vi "Cal Interpolation_3.vi"() -> ()   [LabVIEW 2018]
doc: "This example shows the operation of the 1D interpolation VI using three selectable test sets."
uses:
  <vilib>/Utility/file.llb/Read From Spreadsheet File (DBL).vi
  <vilib>/gmath/NI_Gmath.lvlib
panel:
  in  "file path (dialog if empty)":path=path "C:/IdtATE/Utilities/Calibration  Files/MIXER_TEST_032411_1939.csv"
  in  "y":dbl=201.0
  in  "all rows":dbl[][](array[numeric])=[[50000000.0, 100000000.0, 150000000.0, 200000000.0, 250000000.0, 300000000.0, 350000000.0, 400000000.0, 450000000.0, 500000000.0, 550000000.0, 600000000.0, 650000000.0, 700000000.0, 750000000.0, 800000000.0, 850000000.0, 900000000.0, 950000000.0, 1000000000.0, 1050000000.0, 1100000000.0, 1150000000.0, 1200000000.0, 1250000000.0, 1300000000.0, 1350000000.0, 1400000000.0, 1450000000.0, 1500000000.0, 1550000000.0, 1600000000.0, 1650000000.0, 1700000000.0, 1750000000.0, 1800000000.0, 1850000000.0, 1900000000.0, 1950000000.0, 2000000000.0, 2050000000.0, 2100000000.0, 2150000000.0, 2200000000.0, 2250000000.0, 2300000000.0, 2350000000.0, 2400000000.0, 2450000000.0, 2500000000.0, 2550000000.0, 2600000000.0, 2650000000.0, 2700000000.0, 2750000000.0, 2800000000.0, 2850000000.0, 2900000000.0, 2950000000.0, 3000000000.0], [-0.08, -0.16, -0.21, -0.23, -0.24, -0.28, -0.3, -0.34, -0.33, -0.31, -0.38, -0.37, -0.42, -0.39, -0.48, -0.41, -0.45, -0.41, -0.46, -0.48, -0.53, -0.57, -0.58, -0.65, -0.6, -0.71, -0.66, -0.77, -0.68, -0.78, -0.76, -0.88, -0.81, -0.83, -0.87, -0.83, -0.97, -0.81, -0.92, -0.79, -1.11, -0.76, -0.94, -0.98, -1.08, -0.9, -0.89, -1.14, -1.07, -1.25, -0.93, -1.25, -0.97, -1.38, -1.03, -1.17, -1.06, -1.21, -1.13, -0.98], [-6.65, -6.76, -6.93, -7.18, -7.18, -7.1, -7.38, -7.15, -7.28, -7.26, -7.24, -7.2, -7.36, -7.25, -7.49, -7.47, -7.53, -7.51, -7.88, -7.68, -7.97, -7.71, -7.89, -7.81, -7.91, -7.86, -7.94, -7.9, -7.97, -8.04, -8.08, -8.0, -8.12, -8.12, -8.29, -8.21, -8.41, -8.33, -8.43, -8.28, -8.91, -8.32, -8.78, -8.53, -8.99, -8.69, -8.98, -8.66, -9.24, -8.98, -8.95, -9.08, -9.02, -9.57, -9.73, -10.52, -10.26, -12.76, -13.4, -16.45], [-6.86, -6.86, -6.91, -7.31, -7.13, -7.12, -7.41, -7.13, -7.26, -7.16, -7.21, -7.16, -7.28, -7.19, -7.36, -7.35, -7.47, -7.41, -7.71, -7.57, -7.84, -7.64, -7.81, -7.77, -7.76, -7.89, -7.87, -7.94, -7.84, -8.05, -8.02, -8.06, -8.05, -8.14, -8.3, -8.19, -8.41, -8.36, -8.48, -8.27, -8.95, -8.31, -8.81, -8.49, -8.91, -8.64, -8.83, -8.49, -9.03, -8.8, -8.69, -8.97, -8.8, -9.38, -9.57, -10.78, -10.64, -12.82, -14.4, -17.28], [-0.19, -0.304, -0.304, -0.351, -0.339, -0.296, -0.371, -0.336, -0.432, -0.473, -0.503, -0.432, -0.446, -0.458, -0.627, -0.623, -0.587, -0.637, -0.778, -0.751, -0.707, -0.637, -0.654, -0.623, -0.707, -0.721, -0.778, -0.694, -0.707, -0.821, -0.991, -0.963, -0.778, -0.666, -0.749, -0.963, -1.093, -0.934, -0.877, -0.877, -1.05, -1.056, -0.892, -0.764, -0.877, -1.124, -1.272, -1.166, -1.05, -1.006, -1.008, -1.256, -1.345, -1.05, -1.008, -1.333, -1.516, -1.087, -1.124, -1.331]]
  in  "Freq Select":dbl=41000000.0
  out "Last Ofs Value":dbl=-0.07
  out "Next Ofs Value":dbl=-0.09
  out "Orig Ofs Data":dbl[](array[numeric])=[-0.07, -0.09, -0.13, -0.11, -0.14, -0.19, -0.14, -0.13, -0.21, -0.17, -0.19, -0.24, -0.26, -0.23, -0.25, -0.32, -0.32, -0.31, -0.3, -0.26, -0.27, -0.3, -0.28, -0.25, -0.34, -0.37, -0.34, -0.33, -0.35, -0.31, -0.36, -0.42, -0.36, -0.35, -0.42, -0.46, -0.39, -0.39, -0.39, -0.33, -0.35, -0.42, -0.39, -0.37, -0.39, -0.39, -0.36, -0.41, -0.46, -0.45, -0.48, -0.51, -0.54, -0.53, -0.52, -0.54, -0.53, -0.6, -0.6, -0.52, -0.59, -0.61, -0.57, -0.65, -0.67, -0.62, -0.61, -0.65, -0.68, -0.62, -0.67, -0.68, -0.66, -0.74, -0.78, -0.71, -0.69, -0.74, -0.77, -0.75, -0.8, -0.76, -0.73, -0.82, -0.84, -0.79, -0.74, -0.75, -0.75, -0.8, -0.9, -0.87, -0.74, -0.81, -0.83, -0.79, -0.81, -0.77, -0.74, -0.81, -0.92, -0.87, -0.73, -0.78, -0.81, -0.8, -0.94, -0.92, -0.82, -0.8, -0.9, -0.88, -0.82, -0.87, -0.83, -0.81, -1.01, -0.98, -0.89, -0.91, -1.0, -1.01, -1.03, -1.1, -0.96, -0.88, -1.01, -1.04, -0.98, -1.0, -0.98, -0.97, -1.06, -1.24, -1.07, -0.87, -0.98, -1.04, -1.01, -1.0, -0.95, -0.9, -1.04, -1.22, -1.09, -0.89, -1.01, -0.99, -1.0]
  out "Next Freq Value":dbl=60000000.0
  out "Last Freq Value":dbl=40000000.0
  out "Orig Freq data":dbl[](array[numeric])=[40000000.0, 60000000.0, 80000000.0, 100000000.0, 120000000.0, 140000000.0, 160000000.0, 180000000.0, 200000000.0, 220000000.0, 240000000.0, 260000000.0, 280000000.0, 300000000.0, 320000000.0, 340000000.0, 360000000.0, 380000000.0, 400000000.0, 420000000.0, 440000000.0, 460000000.0, 480000000.0, 500000000.0, 520000000.0, 540000000.0, 560000000.0, 580000000.0, 600000000.0, 620000000.0, 640000000.0, 660000000.0, 680000000.0, 700000000.0, 720000000.0, 740000000.0, 760000000.0, 780000000.0, 800000000.0, 820000000.0, 840000000.0, 860000000.0, 880000000.0, 900000000.0, 920000000.0, 940000000.0, 960000000.0, 980000000.0, 1000000000.0, 1020000000.0, 1040000000.0, 1060000000.0, 1080000000.0, 1100000000.0, 1120000000.0, 1140000000.0, 1160000000.0, 1180000000.0, 1200000000.0, 1220000000.0, 1240000000.0, 1260000000.0, 1280000000.0, 1300000000.0, 1320000000.0, 1340000000.0, 1360000000.0, 1380000000.0, 1400000000.0, 1420000000.0, 1440000000.0, 1460000000.0, 1480000000.0, 1500000000.0, 1520000000.0, 1540000000.0, 1560000000.0, 1580000000.0, 1600000000.0, 1620000000.0, 1640000000.0, 1660000000.0, 1680000000.0, 1700000000.0, 1720000000.0, 1740000000.0, 1760000000.0, 1780000000.0, 1800000000.0, 1820000000.0, 1840000000.0, 1860000000.0, 1880000000.0, 1900000000.0, 1920000000.0, 1940000000.0, 1960000000.0, 1980000000.0, 2000000000.0, 2020000000.0, 2040000000.0, 2060000000.0, 2080000000.0, 2100000000.0, 2120000000.0, 2140000000.0, 2160000000.0, 2180000000.0, 2200000000.0, 2220000000.0, 2240000000.0, 2260000000.0, 2280000000.0, 2300000000.0, 2320000000.0, 2340000000.0, 2360000000.0, 2380000000.0, 2400000000.0, 2420000000.0, 2440000000.0, 2460000000.0, 2480000000.0, 2500000000.0, 2520000000.0, 2540000000.0, 2560000000.0, 2580000000.0, 2600000000.0, 2620000000.0, 2640000000.0, 2660000000.0, 2680000000.0, 2700000000.0, 2720000000.0, 2740000000.0, 2760000000.0, 2780000000.0, 2800000000.0, 2820000000.0, 2840000000.0, 2860000000.0, 2880000000.0, 2900000000.0, 2920000000.0, 2940000000.0, 2960000000.0, 2980000000.0, 3000000000.0]
  out "size(s)":i32[](array[numeric])=[202, 2]
  in  "INst":i32(ring)=1 items=["Sig Gen 3"=1, "Sig Gen 1"=2, "Sig Gen 2"=3, "Spec An"=4, "RF Thru"=5, "IF Thru"=6]
  in  "Tab Control":enum32{"Graph", "Data"}(tab)
  out "1D Interpolation Graph":cluster{"yi":dbl[], "ramp data":dbl[]}[](graph)=[{"yi"=[40000000.0, 60000000.0], "ramp data"=[-0.07, -0.09]}, {"yi"=array[202 elements], "ramp data"=array[202 elements]}]
  out "Interpolated Data":dbl[][](array[numeric])=[[40000000.0, -0.07], [40099502.48756219, -0.07009950248756219], [40199004.97512438, -0.0701990049751244], [40298507.46268657, -0.07029850746268658], [40398009.950248756, -0.07039800995024877], [40497512.43781094, -0.07049751243781095], [40597014.92537314, -0.07059701492537314], [40696517.412935324, -0.07069651741293533], [40796019.90049751, -0.07079601990049751], [40895522.3880597, -0.0708955223880597], [40995024.87562189, -0.0709950248756219], [41094527.36318408, -0.07109452736318408], [41194029.85074627, -0.07119402985074627], [41293532.33830846, -0.07129353233830847], [41393034.82587065, -0.07139303482587066], [41492537.313432835, -0.07149253731343284], [41592039.80099502, -0.07159203980099503], [41691542.28855722, -0.07169154228855722], [41791044.7761194, -0.0717910447761194], [41890547.26368159, -0.07189054726368159], [41990049.75124378, -0.07199004975124379], [42089552.23880597, -0.07208955223880598], [42189054.72636816, -0.07218905472636816], [42288557.213930346, -0.07228855721393035], [42388059.70149254, -0.07238805970149255], [42487562.18905473, -0.07248756218905474], [42587064.676616915, -0.07258706467661692], [42686567.1641791, -0.07268656716417911], [42786069.651741296, -0.0727860696517413], [42885572.13930348, -0.0728855721393035], [42985074.62686567, -0.07298507462686568], [43084577.114427865, -0.07308457711442787], [43184079.60199005, -0.07318407960199005], [43283582.08955224, -0.07328358208955224], [43383084.577114426, -0.07338308457711443], [43482587.06467662, -0.07348258706467663], [43582089.55223881, -0.07358208955223881], [43681592.039800994, -0.073681592039801], [43781094.52736318, -0.07378109452736319], [43880597.014925376, -0.07388059701492539], [43980099.50248756, -0.07398009950248757], [44079601.99004975, -0.07407960199004976], [44179104.477611944, -0.07417910447761195], [44278606.96517413, -0.07427860696517413], [44378109.45273632, -0.07437810945273632], [44477611.940298505, -0.0744776119402985], [44577114.4278607, -0.0745771144278607], [44676616.91542289, -0.07467661691542289], [44776119.40298507, -0.07477611940298508], [44875621.89054726, -0.07487562189054726], [44975124.378109455, -0.07497512437810946], [45074626.86567164, -0.07507462686567165], [45174129.35323383, -0.07517412935323384], [45273631.84079602, -0.07527363184079602], [45373134.32835821, -0.07537313432835821], [45472636.8159204, -0.0754726368159204], [45572139.303482585, -0.07557213930348258], [45671641.79104478, -0.07567164179104478], [45771144.278606966, -0.07577114427860697], [45870646.76616915, -0.07587064676616916], [45970149.25373134, -0.07597014925373134], [46069651.741293535, -0.07606965174129354], [46169154.22885572, -0.07616915422885573], [46268656.71641791, -0.07626865671641792], [46368159.2039801, -0.0763681592039801], [46467661.69154229, -0.07646766169154229], [46567164.17910448, -0.07656716417910447], [46666666.666666664, -0.07666666666666666], [46766169.15422886, -0.07676616915422886], [46865671.641791046, -0.07686567164179105], [46965174.12935323, -0.07696517412935323], [47064676.61691542, -0.07706467661691542], [47164179.104477614, -0.07716417910447762], [47263681.5920398, -0.0772636815920398], [47363184.07960199, -0.077363184079602], [47462686.56716418, -0.07746268656716418], [47562189.05472637, -0.07756218905472637], [47661691.54228856, -0.07766169154228857], [47761194.02985074, -0.07776119402985075], [47860696.51741294, -0.07786069651741294], [47960199.004975125, -0.07796019900497513], [48059701.49253731, -0.07805970149253731], [48159203.9800995, -0.0781592039800995], [48258706.46766169, -0.0782587064676617], [48358208.95522388, -0.07835820895522388], [48457711.44278607, -0.07845771144278607], [48557213.93034826, -0.07855721393034826], [48656716.41791045, -0.07865671641791046], [48756218.905472636, -0.07875621890547264], [48855721.39303482, -0.07885572139303483], [48955223.88059701, -0.07895522388059702], [49054726.368159205, -0.0790547263681592], [49154228.85572139, -0.07915422885572139], [49253731.34328358, -0.07925373134328358], [49353233.83084577, -0.07935323383084578], [49452736.31840796, -0.07945273631840796], [49552238.80597015, -0.07955223880597015], [49651741.29353234, -0.07965174129353235], [49751243.78109453, -0.07975124378109454], [49850746.268656716, -0.07985074626865672], [49950248.7562189, -0.07995024875621891], [50049751.24378109, -0.0800497512437811], [50149253.731343284, -0.08014925373134328], [50248756.21890547, -0.08024875621890547], [50348258.70646766, -0.08034825870646765], [50447761.19402985, -0.08044776119402985], [50547263.68159204, -0.08054726368159204], [50646766.16915423, -0.08064676616915423], [50746268.65671642, -0.08074626865671643], [50845771.14427861, -0.08084577114427861], [50945273.631840795, -0.0809452736318408], [51044776.11940298, -0.08104477611940299], [51144278.60696517, -0.08114427860696517], [51243781.094527364, -0.08124378109452736], [51343283.58208955, -0.08134328358208956], [51442786.06965174, -0.08144278606965175], [51542288.55721393, -0.08154228855721393], [51641791.04477612, -0.08164179104477612], [51741293.53233831, -0.0817412935323383], [51840796.0199005, -0.0818407960199005], [51940298.50746269, -0.08194029850746269], [52039800.995024875, -0.08203980099502488], [52139303.48258706, -0.08213930348258706], [52238805.97014926, -0.08223880597014925], [52338308.45771144, -0.08233830845771145], [52437810.94527363, -0.08243781094527364], [52537313.43283582, -0.08253731343283582], [52636815.92039801, -0.08263681592039801], [52736318.4079602, -0.0827363184079602], [52835820.895522386, -0.08283582089552238], [52935323.38308458, -0.08293532338308458], [53034825.87064677, -0.08303482587064677], [53134328.358208954, -0.08313432835820896], [53233830.84577114, -0.08323383084577114], [53333333.333333336, -0.08333333333333333], [53432835.82089552, -0.08343283582089553], [53532338.30845771, -0.08353233830845772], [53631840.7960199, -0.0836318407960199], [53731343.28358209, -0.08373134328358209], [53830845.77114428, -0.08383084577114427], [53930348.258706465, -0.08393034825870646], [54029850.74626866, -0.08402985074626866], [54129353.23383085, -0.08412935323383085], [54228855.721393034, -0.08422885572139303], [54328358.20895523, -0.08432835820895522], [54427860.696517415, -0.08442786069651742], [54527363.1840796, -0.0845273631840796], [54626865.67164179, -0.0846268656716418], [54726368.15920398, -0.08472636815920398], [54825870.64676617, -0.08482587064676617], [54925373.13432836, -0.08492537313432835], [55024875.621890545, -0.08502487562189054], [55124378.10945274, -0.08512437810945274], [55223880.59701493, -0.08522388059701493], [55323383.08457711, -0.08532338308457711], [55422885.57213931, -0.08542288557213931], [55522388.059701495, -0.0855223880597015], [55621890.54726368, -0.08562189054726368], [55721393.03482587, -0.08572139303482587], [55820895.522388056, -0.08582089552238806], [55920398.00995025, -0.08592039800995024], [56019900.49751244, -0.08601990049751243], [56119402.985074624, -0.08611940298507462], [56218905.47263682, -0.08621890547263682], [56318407.960199006, -0.086318407960199], [56417910.44776119, -0.08641791044776119], [56517412.93532339, -0.08651741293532339], [56616915.422885574, -0.08661691542288558], [56716417.91044776, -0.08671641791044776], [56815920.39800995, -0.08681592039800995], [56915422.885572135, -0.08691542288557214], [57014925.37313433, -0.08701492537313434], [57114427.86069652, -0.08711442786069652], [57213930.348258704, -0.0872139303482587], [57313432.8358209, -0.0873134328358209], [57412935.323383085, -0.08741293532338308], [57512437.81094527, -0.08751243781094527], [57611940.29850747, -0.08761194029850747], [57711442.78606965, -0.08771144278606964], [57810945.27363184, -0.08781094527363184], [57910447.76119403, -0.08791044776119403], [58009950.248756215, -0.08800995024875621], [58109452.73631841, -0.08810945273631841], [58208955.2238806, -0.0882089552238806], [58308457.71144278, -0.08830845771144279], [58407960.19900498, -0.08840796019900497], [58507462.686567165, -0.08850746268656716], [58606965.17412935, -0.08860696517412935], [58706467.66169155, -0.08870646766169155], [58805970.149253726, -0.08880597014925372], [58905472.63681592, -0.08890547263681592], [59004975.12437811, -0.0890049751243781], [59104477.611940295, -0.08910447761194029], [59203980.09950249, -0.08920398009950249], [59303482.587064676, -0.08930348258706468], [59402985.07462686, -0.08940298507462686], [59502487.56218906, -0.08950248756218905], [59601990.049751244, -0.08960199004975124], [59701492.53731343, -0.08970149253731342], [59800995.024875626, -0.08980099502487562], [59900497.512437806, -0.0899004975124378], [60000000.0, -0.09]]
  out "Original Data":dbl[][](array[numeric])=[[40000000.0, -0.07], [60000000.0, -0.09]]
  # "294976"
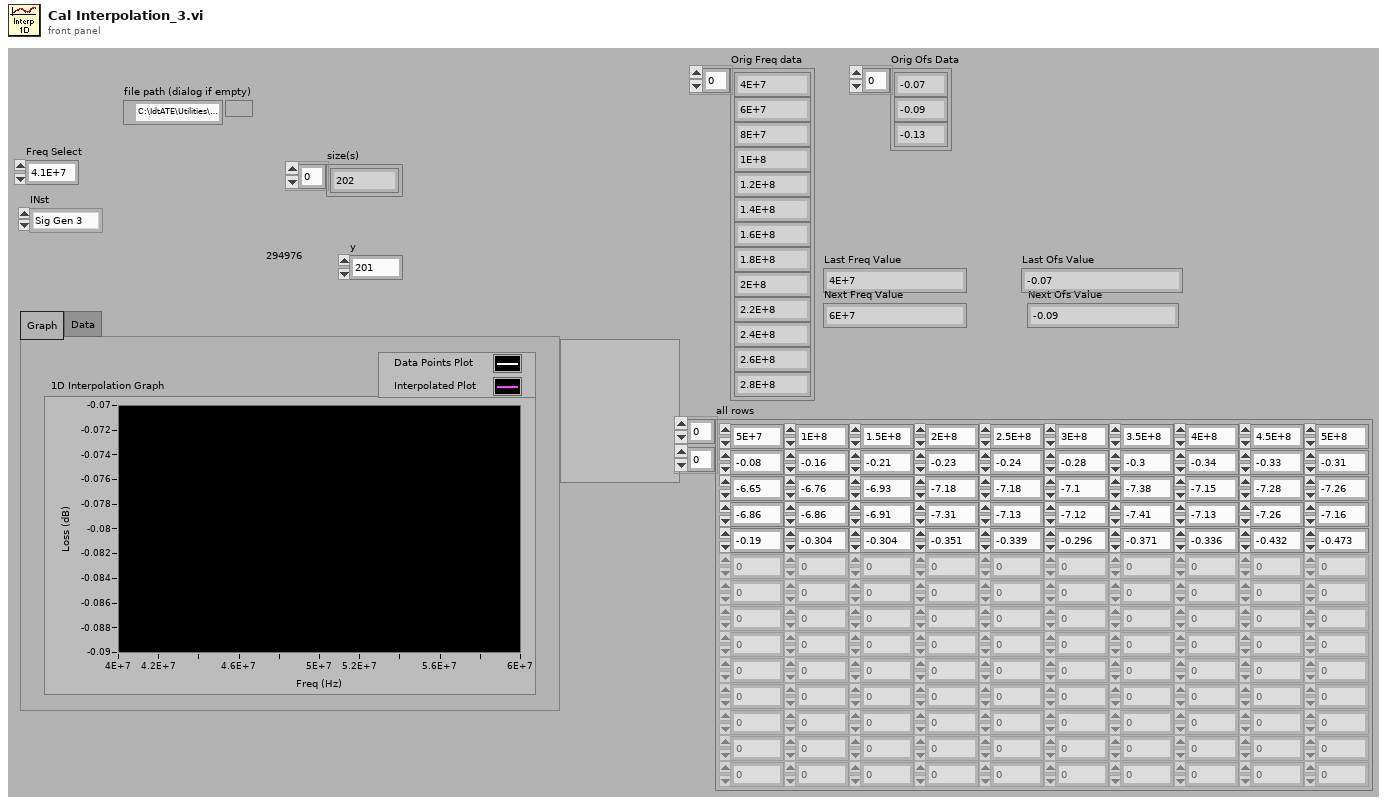
[diagram p1: front panel]
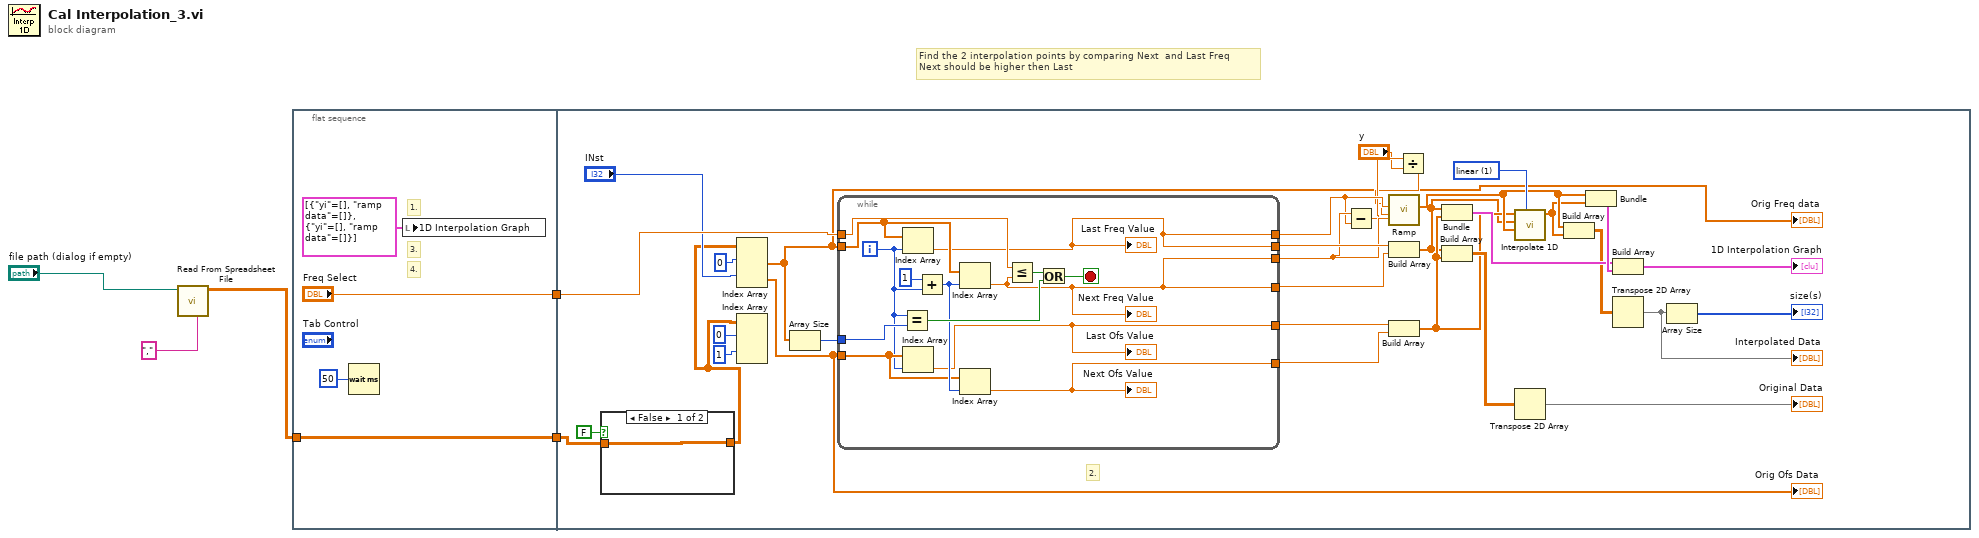
[diagram p0: block diagram]
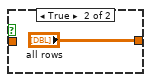
[diagram p2: hidden frame]
diagram:
  # "Find the 2 interpolation points by comparing Next  and Last Freq\nNext should be higher then Last"
  n1 = call-poly <vilib>:"Read From Spreadsheet File.vi"("delimiter (\\t)"="," ("delimiter (\\t)"), "file path (dialog if empty)"="file path (dialog if empty)") -> ("all rows"=w1:dbl[][])  [unwired: 5 in, 4 out]
  n2 = flat-sequence {
    tunnel: ["Freq Select"] -> w5
    tunnel: [w6] -> w2
    tunnel: w1 -> [w6]
    tunnel: w5 -> [w22]
    tunnel: w2 -> [w11]
    frame #0 {
      # "4."
      # "3."
      # "1."
      n3 = Wait (ms)(milliseconds to wait=u32 50) -> ()  [unwired: 1 out]
      n4 = local write "1D Interpolation Graph"(cluster{"yi":i32[], "ramp data":i32[]}[] [{"yi"=[], "ramp data"=[]}, {"yi"=[], "ramp data"=[]}] ("1D Interpolation Graph")) -> ()
    }
    frame #1 {
      w38 = 1 items=["nearest", "linear", "spline", "cubic Hermite", "Lagrange"] ("Method")
      # "2."
      n5 = case shown="False" FALSE {
        tunnel: [w43 "all rows"] -> w12
        tunnel: w11 -> [w43 _]
        frame False {
        }
        frame True {
        }
      }
      n6 = Index Array(array=w12, index (row) #1=0 ("index (row)"), index (row) #2="INst") -> (element #1=w15:dbl[], element #2=w16:dbl[])  [unwired: 2 in]
      "Orig Freq data" <- w15
      "Orig Ofs Data" <- w16
      n7 = Index Array(array=w12, index (row) #1=0 ("index (row)"), index (row) #2=1 ("index (row)")) -> ()  [unwired: 2 in, 2 out]
      n8 = Array Size(array=w15) -> (size(s)=w41:i32)
      n9 = while {
        tunnel: w15 -> [w57]
        tunnel: w41 -> [w56]
        tunnel: w22 -> [w55]
        tunnel: [w46] -> w40
        tunnel: [w45] -> w39
        tunnel: w16 -> [w50]
        tunnel: [w48] -> w26
        tunnel: [w47] -> w25
        tunnel: [w46] -> w20
        tunnel: [w45] -> w21
        i -> [w49]
        stop <- w53 stop-if-true
        n10 = Equal?(x=w49, y=w56) -> (x = y?=w54:bool)
        n11 = Index Array(array=w57, index=w49) -> (element=w46:dbl)
        "Last Freq Value" <- w46
        n12 = Index Array(array=w50, index=w49) -> (element=w48:dbl)
        "Last Ofs Value" <- w48
        n13 = Add(x=1, y=w49) -> (x+y=w51:i32)
        n14 = Index Array(array=w57, index=w51) -> (element=w45:dbl)
        "Next Freq Value" <- w45
        n15 = Index Array(array=w50, index=w51) -> (element=w47:dbl)
        "Next Ofs Value" <- w47
        n16 = Less Or Equal?(x=w55, y=w45) -> (x <= y?=w52:bool)
        n17 = Or(x=w52, y=w54) -> (x .or. y?=w53:bool)
      }
      n18 = Subtract(x=w21, y=w20) -> (x-y=w19:dbl)
      n19 = Build Array(w40, w39) -> (w23:dbl[])
      n20 = Build Array(w26, w25) -> (w24:dbl[])
      n21 = Divide(x=w19, y="y") -> (x/y=w17:dbl)
      n22 = call "Ramp.vi"("# of Samples"=w21, "Start"=w17, "Stop"=w20) -> ("Output"=w31:dbl[])  [unwired: 8 in]
      n23 = Bundle(w23, w24) -> (w35:cluster{dbl[], dbl[]})  [unwired: 1 in]
      n24 = Build Array(w23, w24) -> (w34:dbl[][])
      n25 = call <vilib>:"Interpolate 1D.vi"("method"=w38, "xi"=w31, "X"=w23, "Y"=w24) -> ("yi"=w30:dbl[])  [unwired: 5 in, 2 out]
      n26 = Transpose 2D Array(2D array=w34) -> (transposed array=→"Original Data":dbl[][])
      n27 = Build Array(w31, w30) -> (w32:dbl[][])
      n28 = Bundle("Output"=w31, "yi"=w30) -> (w36:cluster{"Output":dbl[], "yi":dbl[]})  [unwired: 1 in]
      n29 = Build Array(w35, w36) -> (→"1D Interpolation Graph":cluster{"Output":dbl[], "yi":dbl[]}[])
      n30 = Transpose 2D Array(2D array=w32) -> (transposed array=w29:dbl[][])
      "Interpolated Data" <- w29
      n31 = Array Size(array=w29) -> (size(s)=→"size(s)":i32[])
    }
  }
